vi "getConfigurations.vi"(0 "Device In":T1={"Date"="", "On-Nonce"="", "eid"="990ec2d1208dce12e8c8d73d", "wid"="2816a0ac3f158e698c5324a2", "did"="78f5bf641b1754cc5a2885a6", "name"="", "method"="", "Accept"="", "User-Agent"="", "Content-Type"="", "stack"="", "headers"=[], "payload"="", "addition"="", "path"="", "Authorization"="", "secret_key"="", "access_key"=""}, 11 "error in":errorcluster) -> (4 "Device Out":T1={"Date"="Thu, 16 Apr 2020 23:19:12 GMT", "On-Nonce"="nlS7Y9rr4jS35A8DK9B3OToU", "eid"="990ec2d1208dce12e8c8d73d", "wid"="2816a0ac3f158e698c5324a2", "did"="78f5bf641b1754cc5a2885a6", "name"="", "method"="get", "Accept"="", "User-Agent"="", "Content-Type"="", "stack"="https://rogers.onshape.com", "headers"=["Content-Type:application/json", "Date:Thu, 16 Apr 2020 23:19:12 GMT", "On-Nonce:nlS7Y9rr4jS35A8DK9B3OToU", "Authorization:On 5WRzTWmAmwc94xTxHfKZAg5i:HmacSHA256:lDyQC1x2JlGNCtdzVGE5L8N41PUpGQIlxBBiesg5jjs=", "User_agent:Onshape Python Sample App", "Accept:application/json"], "payload"="", "addition"="application/json", "path"="/api/partstudios/d/78f5bf641b1754cc5a2885a6/w/2816a0ac3f158e698c5324a2/e/990ec2d1208dce12e8c8d73d/sketches", "Authorization"="On 5WRzTWmAmwc94xTxHfKZAg5i:HmacSHA256:lDyQC1x2JlGNCtdzVGE5L8N41PUpGQIlxBBiesg5jjs=", "secret_key"="oi7XeQrYfdCYv3AKwLnpJCWbiY7ldMXDXqIW5a1h4ENYmHDu", "access_key"="5WRzTWmAmwc94xTxHfKZAg5i"}, 6 "Comm":T2={"url"="https://rogers.onshape.com/api/partstudios/d/78f5bf641b1754cc5a2885a6/w/2816a0ac3f158e698c5324a2/e/990ec2d1208dce12e8c8d73d/sketches?", "sent headers"="Accept: application/json\r\nAuthorization: On 5WRzTWmAmwc94xTxHfKZAg5i:HmacSHA256:lDyQC1x2JlGNCtdzVGE5L8N41PUpGQIlxBBiesg5jjs=\r\nContent-Type: application/json\r\nDate: Thu, 16 Apr 2020 23:19:12 GMT\r\nOn-Nonce: nlS7Y9rr4jS35A8DK9B3OToU\r\nUser_agent: Onshape Python Sample App", "sent body"="", "headers"="HTTP/1.1 200 OK\r\nServer: nginx\r\nDate: Thu, 16 Apr 2020 23:19:12 GMT\r\nContent-Type: application/json;charset=UTF-8;qs=0.9\r\nContent-Length: 2372\r\nConnection: keep-alive\r\nVary: Accept-Encoding\r\nOn-Version: 1.111.25149.0c1f2eb083aa\r\nOn-Request-Id: a78cc699fde7b461387b36e3\r\nDeprecation: version=UNDEFINED, message=\"You specified mediatype application/json;charset=UTF-8;qs=0.9 and this endpoint will currently accept application/vnd.onshape.v1+json;charset=UTF-8;qs=0.1. Please consider updating to the latest version by specifying application/vnd.onshape.v1+json;charset=UTF-8;qs=0.1 within the Accept header.\r\nSet-Cookie: _u=webservice-3e25a82e; Path=/; Secure; HttpOnly;\r\nX-Frame-Options: SAMEORIGIN\r\nStrict-Transport-Security: max-age=31536000; includeSubDomains\r\nX-Content-Type-Options: nosniff\r\nX-XSS-Protection: 1; mode=block\r\nContent-Security-Policy-Report-Only: object-src 'self' https://embedwistia-a.akamaihd.net; report-uri /api/csp\r\n\r\n", "body"="{\n  \"sketches\" : [ {\n    \"sketch\" : \"Sketch 1\",\n    \"featureId\" : \"FbqM6rYzUBbMRp8_0\",\n    \"transformMatrix\" : [ 1.0, 0.0, 0.0, 0.0, 0.0, 1.0, 0.0, 0.0, 0.0, 0.0, 1.0, 0.0, 0.0, 0.0, 0.0, 1.0 ],\n    \"featuresUsed\" : [ ],\n    \"geomEntities\" : [ {\n      \"id\" : \"C471k0qsEi0Q.start\",\n      \"entityType\" : \"point\",\n      \"point\" : [ 0.017283352091908455, -0.007151731755584478 ]\n    }, {\n      \"id\" : \"C471k0qsEi0Q.end\",\n      \"entityType\" : \"point\",\n      \"point\" : [ -0.04529430344700813, 0.05423396825790405 ]\n    }, {\n      \"id\" : \"C471k0qsEi0Q.0.internal\",\n      \"entityType\" : \"point\",\n      \"point\" : [ 0.017283352091908455, -0.007151731755584478 ]\n    }, {\n      \"id\" : \"C471k0qsEi0Q.1.internal\",\n      \"entityType\" : \"point\",\n      \"point\" : [ 0.05095608904957771, 0.022945139557123184 ]\n    }, {\n      \"id\" : \"C471k0qsEi0Q.2.internal\",\n      \"entityType\" : \"point\",\n      \"point\" : [ 0.02443508431315422, 0.05780983343720436 ]\n    }, {\n      \"id\" : \"C471k0qsEi0Q.3.internal\",\n      \"entityType\" : \"point\",\n      \"point\" : [ -0.018177319318056107, 0.039334528148174286 ]\n    }, {\n      \"id\" : \"C471k0qsEi0Q.4.internal\",\n      \"entityType\" : \"point\",\n      \"point\" : [ -0.04529430344700813, 0.05423396825790405 ]\n    }, {\n      \"id\" : \"C471k0qsEi0Q.startDerivative\",\n      \"entityType\" : \"point\",\n      \"point\" : [ 0.03353424071398461, 8.902966705931049E-4 ],\n      \"isConstruction\" : true\n    }, {\n      \"id\" : \"C471k0qsEi0Q.endDerivative\",\n      \"entityType\" : \"point\",\n      \"point\" : [ -0.0368764138795279, 0.04584760236142172 ],\n      \"isConstruction\" : true\n    }, {\n      \"id\" : \"C471k0qsEi0Q\",\n      \"entityType\" : \"interpolatedSplineSegment\",\n      \"periodic\" : false,\n      \"startHandle\" : [ 0.03353424071398461, 8.902966705931043E-4 ],\n      \"endHandle\" : [ -0.03687641387952791, 0.045847602361421734 ],\n      \"startDerivative\" : [ 0.18655982097041743, 0.0923222980796617 ],\n      \"endDerivative\" : [ -0.1167534466674709, 0.11631622339302505 ],\n      \"interpolationPoints\" : [ [ 0.017283352091908455, -0.007151731755584478 ], [ 0.05095608904957771, 0.022945139557123184 ], [ 0.02443508431315422, 0.05780983343720436 ], [ -0.018177319318056107, 0.039334528148174286 ], [ -0.04529430344700813, 0.05423396825790405 ] ],\n      \"startParameter\" : 0.0,\n      \"endParameter\" : 1.0,\n      \"endPointIds\" : [ \"C471k0qsEi0Q.start\", \"C471k0qsEi0Q.end\" ]\n    } ]\n  } ]\n}", "Sent"="get https://rogers.onshape.com/api/partstudios/d/78f5bf641b1754cc5a2885a6/w/2816a0ac3f158e698c5324a2/e/990ec2d1208dce12e8c8d73d/sketches? \n\nAccept: application/json\r\nAuthorization: On 5WRzTWmAmwc94xTxHfKZAg5i:HmacSHA256:lDyQC1x2JlGNCtdzVGE5L8N41PUpGQIlxBBiesg5jjs=\r\nContent-Type: application/json\r\nDate: Thu, 16 Apr 2020 23:19:12 GMT\r\nOn-Nonce: nlS7Y9rr4jS35A8DK9B3OToU\r\nUser_agent: Onshape Python Sample App\n\n", "Received"="HTTP/1.1 200 OK\r\nServer: nginx\r\nDate: Thu, 16 Apr 2020 23:19:12 GMT\r\nContent-Type: application/json;charset=UTF-8;qs=0.9\r\nContent-Length: 2372\r\nConnection: keep-alive\r\nVary: Accept-Encoding\r\nOn-Version: 1.111.25149.0c1f2eb083aa\r\nOn-Request-Id: a78cc699fde7b461387b36e3\r\nDeprecation: version=UNDEFINED, message=\"You specified mediatype application/json;charset=UTF-8;qs=0.9 and this endpoint will currently accept application/vnd.onshape.v1+json;charset=UTF-8;qs=0.1. Please consider updating to the latest version by specifying application/vnd.onshape.v1+json;charset=UTF-8;qs=0.1 within the Accept header.\r\nSet-Cookie: _u=webservice-3e25a82e; Path=/; Secure; HttpOnly;\r\nX-Frame-Options: SAMEORIGIN\r\nStrict-Transport-Security: max-age=31536000; includeSubDomains\r\nX-Content-Type-Options: nosniff\r\nX-XSS-Protection: 1; mode=block\r\nContent-Security-Policy-Report-Only: object-src 'self' https://embedwistia-a.akamaihd.net; report-uri /api/csp\r\n\r\n\n\n{\n  \"sketches\" : [ {\n    \"sketch\" : \"Sketch 1\",\n    \"featureId\" : \"FbqM6rYzUBbMRp8_0\",\n    \"transformMatrix\" : [ 1.0, 0.0, 0.0, 0.0, 0.0, 1.0, 0.0, 0.0, 0.0, 0.0, 1.0, 0.0, 0.0, 0.0, 0.0, 1.0 ],\n    \"featuresUsed\" : [ ],\n    \"geomEntities\" : [ {\n      \"id\" : \"C471k0qsEi0Q.start\",\n      \"entityType\" : \"point\",\n      \"point\" : [ 0.017283352091908455, -0.007151731755584478 ]\n    }, {\n      \"id\" : \"C471k0qsEi0Q.end\",\n      \"entityType\" : \"point\",\n      \"point\" : [ -0.04529430344700813, 0.05423396825790405 ]\n    }, {\n      \"id\" : \"C471k0qsEi0Q.0.internal\",\n      \"entityType\" : \"point\",\n      \"point\" : [ 0.017283352091908455, -0.007151731755584478 ]\n    }, {\n      \"id\" : \"C471k0qsEi0Q.1.internal\",\n      \"entityType\" : \"point\",\n      \"point\" : [ 0.05095608904957771, 0.022945139557123184 ]\n    }, {\n      \"id\" : \"C471k0qsEi0Q.2.internal\",\n      \"entityType\" : \"point\",\n      \"point\" : [ 0.02443508431315422, 0.05780983343720436 ]\n    }, {\n      \"id\" : \"C471k0qsEi0Q.3.internal\",\n      \"entityType\" : \"point\",\n      \"point\" : [ -0.018177319318056107, 0.039334528148174286 ]\n    }, {\n      \"id\" : \"C471k0qsEi0Q.4.internal\",\n      \"entityType\" : \"point\",\n      \"point\" : [ -0.04529430344700813, 0.05423396825790405 ]\n    }, {\n      \"id\" : \"C471k0qsEi0Q.startDerivative\",\n      \"entityType\" : \"point\",\n      \"point\" : [ 0.03353424071398461, 8.902966705931049E-4 ],\n      \"isConstruction\" : true\n    }, {\n      \"id\" : \"C471k0qsEi0Q.endDerivative\",\n      \"entityType\" : \"point\",\n      \"point\" : [ -0.0368764138795279, 0.04584760236142172 ],\n      \"isConstruction\" : true\n    }, {\n      \"id\" : \"C471k0qsEi0Q\",\n      \"entityType\" : \"interpolatedSplineSegment\",\n      \"periodic\" : false,\n      \"startHandle\" : [ 0.03353424071398461, 8.902966705931043E-4 ],\n      \"endHandle\" : [ -0.03687641387952791, 0.045847602361421734 ],\n      \"startDerivative\" : [ 0.18655982097041743, 0.0923222980796617 ],\n      \"endDerivative\" : [ -0.1167534466674709, 0.11631622339302505 ],\n      \"interpolationPoints\" : [ [ 0.017283352091908455, -0.007151731755584478 ], [ 0.05095608904957771, 0.022945139557123184 ], [ 0.02443508431315422, 0.05780983343720436 ], [ -0.018177319318056107, 0.039334528148174286 ], [ -0.04529430344700813, 0.05423396825790405 ] ],\n      \"startParameter\" : 0.0,\n      \"endParameter\" : 1.0,\n      \"endPointIds\" : [ \"C471k0qsEi0Q.start\", \"C471k0qsEi0Q.end\" ]\n    } ]\n  } ]\n}"}, 10 "error":i32, 15 "error out":errorcluster)   [LabVIEW 2020]
uses:
  _SubVI/HTTPComm.ctl
  _SubVI/Cluster.ctl
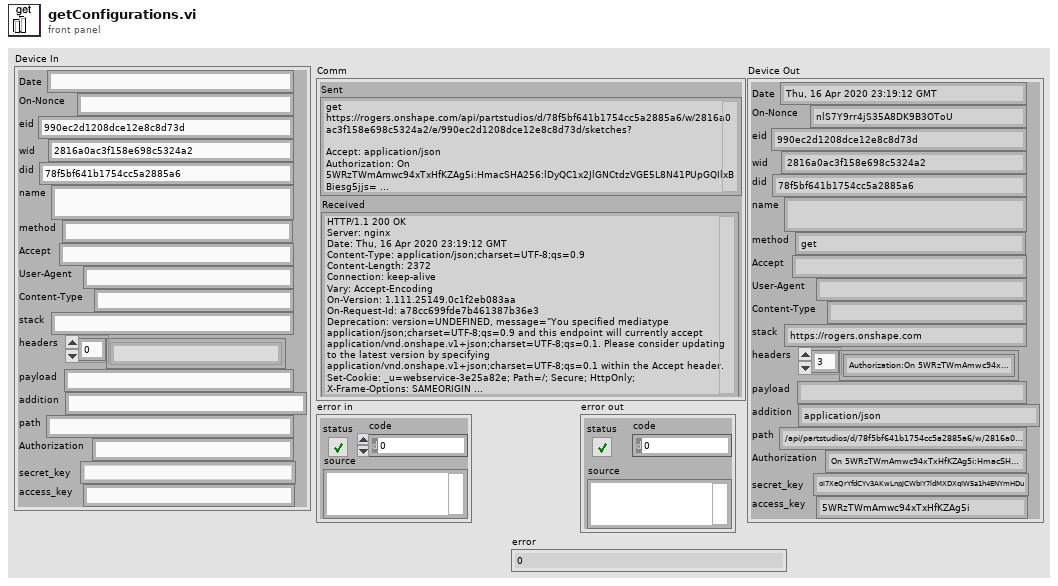
[diagram p1: front panel]
types:
  T1 = typedef "Cluster.ctl" = cluster{"Date":string, "On-Nonce":string, "eid":string, "wid":string, "did":string, "name":string, "method":string, "Accept":string, "User-Agent":string, "Content-Type":string, "stack":string, "headers":string[], "payload":string, "addition":string, "path":string, "Authorization":string, "secret_key":string, "access_key":string}
  T2 = typedef "HTTPComm.ctl" = cluster{"url":string, "sent headers":string, "sent body":string, "headers":string, "body":string, "Sent":string, "Received":string}
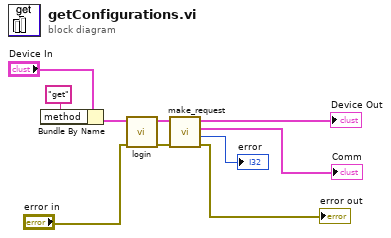
[diagram p0: block diagram]
diagram:
  n1 = Bundle By Name(cluster="Device In", "method"="get" ("Method")) -> (w3:T1)
  n2 = call "login.vi"("error in"="error in", "Device In"=w3) -> ("error out"=w6:errorcluster, "Device Out"=w9:T1)  [unwired: 8 in]
  n3 = call "make_request.vi"("Error in"=w6, "Device In"=w9) -> ("error out"=→"error out":errorcluster, "error"=→"error":i32, "Comm"=→"Comm":T2, "Device Out"=→"Device Out":T1)  [unwired: 6 in]
